vi "Read BMS Status.vi"() -> ()   [LabVIEW 2016]
uses:
  Tests/BMS Status.ctl
  Program Files (x86)/National Instruments/LabVIEW 2016/examples/robotics/EPOS2 CANOpen Driver/Low Level VIs/Typedefs/CAN Refnum.ctl
  Program Files (x86)/National Instruments/LabVIEW 2016/examples/robotics/EPOS2 CANOpen Driver/Low Level VIs/Typedefs/CAN Session Pointer.ctl
  Program Files (x86)/National Instruments/LabVIEW 2016/examples/robotics/EPOS2 CANOpen Driver/Low Level VIs/Typedefs/CAN Communication References.ctl
  Program Files (x86)/National Instruments/LabVIEW 2016/examples/robotics/EPOS2 CANOpen Driver/Low Level VIs/Typedefs/kill process notifier array.ctl
  Program Files (x86)/National Instruments/LabVIEW 2016/examples/robotics/EPOS2 CANOpen Driver/Low Level VIs/Typedefs/Write Queue.ctl
  Program Files (x86)/National Instruments/LabVIEW 2016/examples/robotics/EPOS2 CANOpen Driver/Low Level VIs/Typedefs/FPGA CAN Frame Cluster.ctl
  Read single CAN.vi
  Data to BMS Status.vi
panel:
  out "error out":errorcluster
  out "CAN Session Out":T1
  in  "CAN Session In":T1=refnum
  in  "error in":errorcluster
  in  "timeout in ms (-1)":i32=-1
  out "BMS Status":T2
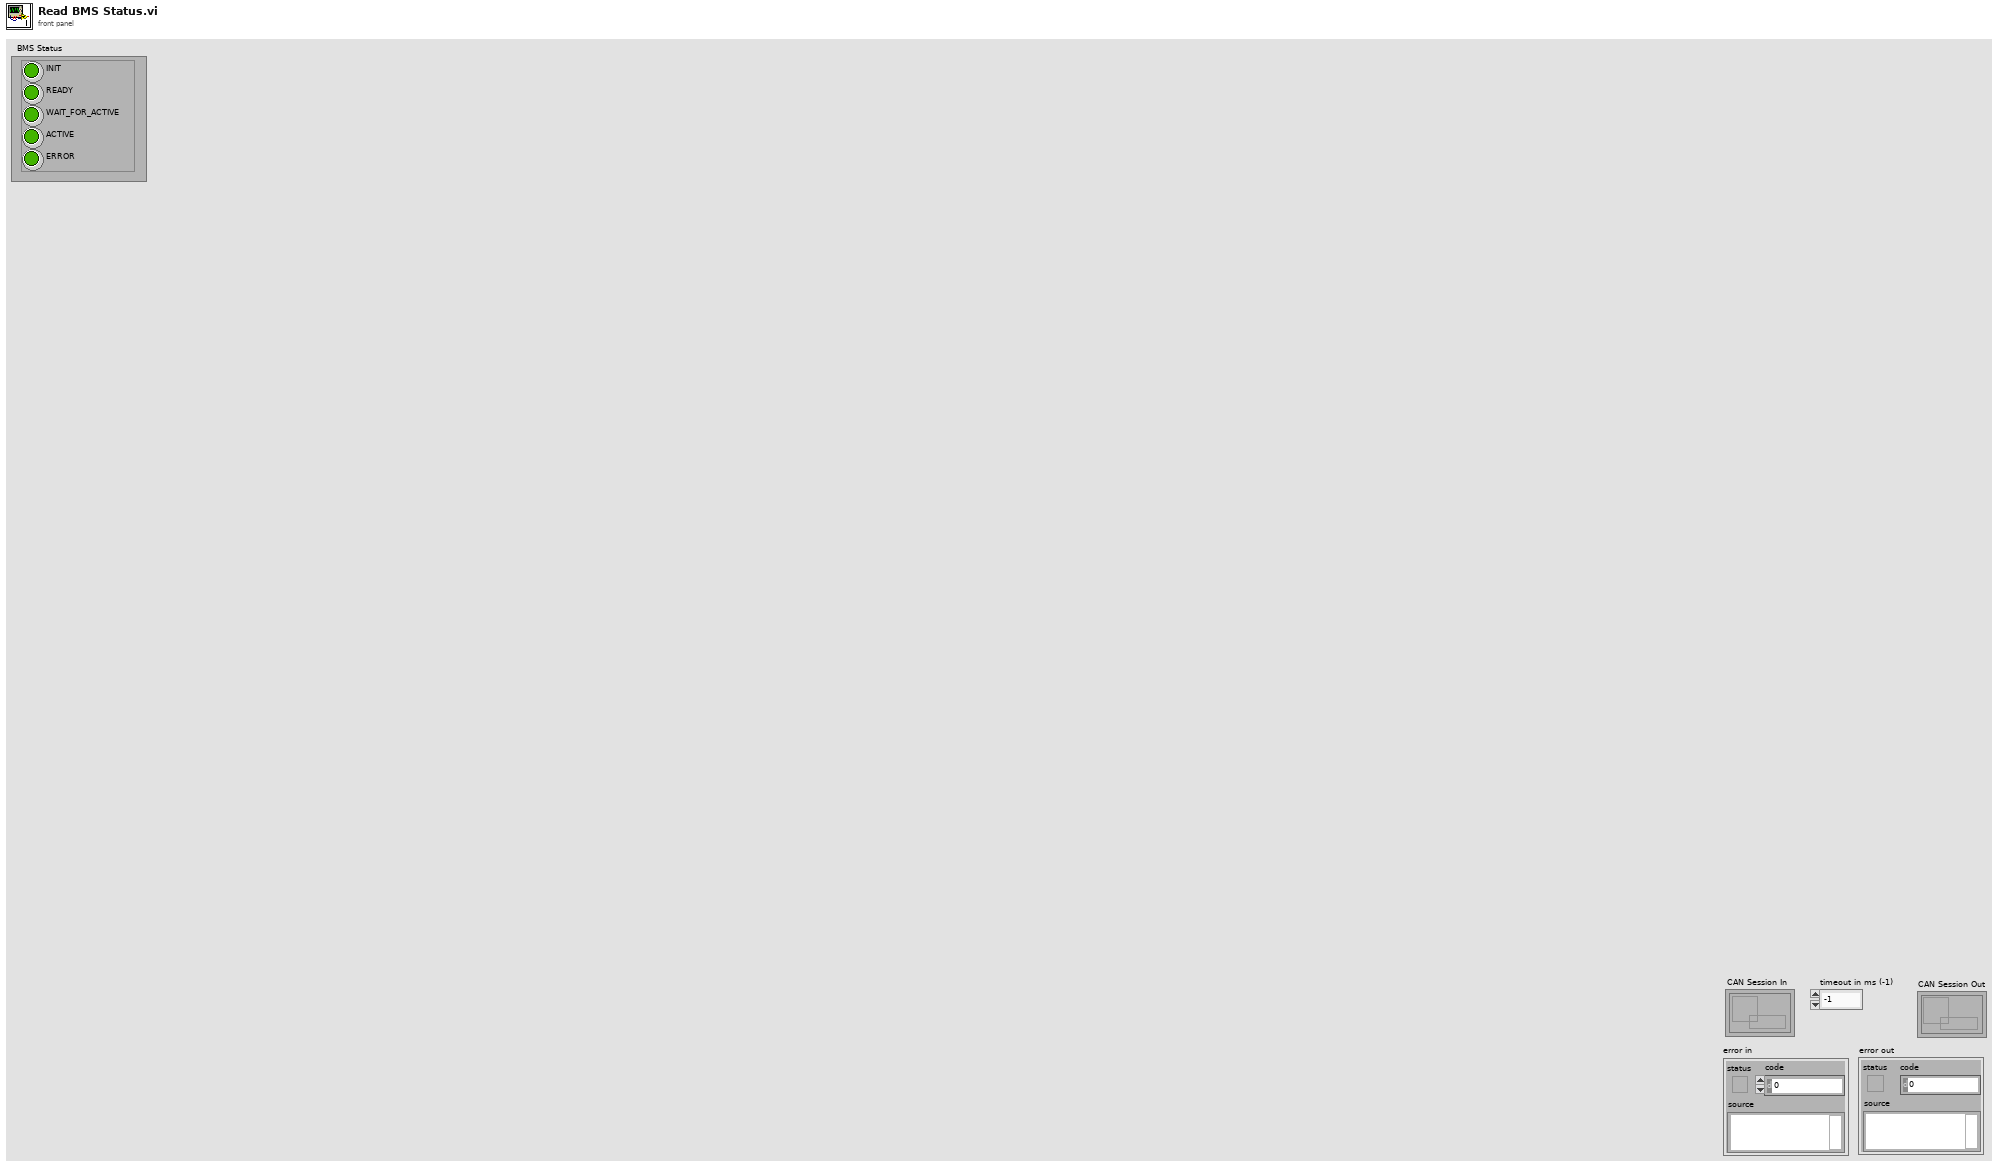
[diagram p1: front panel]
types:
  T1 = typedef "CAN Refnum.ctl" = refnum<k1>
  T2 = typedef "BMS Status.ctl" = cluster{"INIT":bool, "READY":bool, "WAIT_FOR_ACTIVE":bool, "ACTIVE":bool, "ERROR":bool}
  T3 = typedef "FPGA CAN Frame Cluster.ctl" = cluster{"Timestamp":u64, "Identifier":u32, "Type":u8, "InfoA":u8, "InfoB":u8, "DataLength":u8, "Data":u8[]}
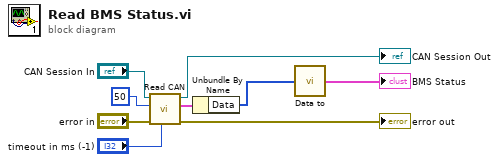
[diagram p0: block diagram]
diagram:
  n1 = call-poly "Read CAN.vi"("timeout in ms (-1)"="timeout in ms (-1)", "error in"="error in", "ID"=50 ("Data 0"), "CAN Session In"="CAN Session In") -> ("error out"=→"error out":errorcluster, "CAN Frame Out"=w9:T3, "CAN Session Out"=→"CAN Session Out":T1)  [unwired: 5 in]
  n2 = Unbundle By Name(w9) -> ("Data"=w8:u8[])
  n3 = call-poly "Data to.vi"("Data"=w8) -> ("BMS Status"=→"BMS Status":T2)
